vi "Write Array of Observer Refnum.vi"(8 "error in (no error)":errorcluster, 10 "Array of Observer Refnum":refnum<vi>, 11 "WT1600 in":refnum<class "WT1600.lvclass">) -> (0 "error out":errorcluster, 3 "WT1600 out":refnum<class "WT1600.lvclass">)   [LabVIEW 2013, in "WT1600.lvlib" / "WT1600.lvclass"]
uses:
  WT1600.lvclass
  <vilib>/ActorFramework/Message Enqueuer/Message Enqueuer.lvclass
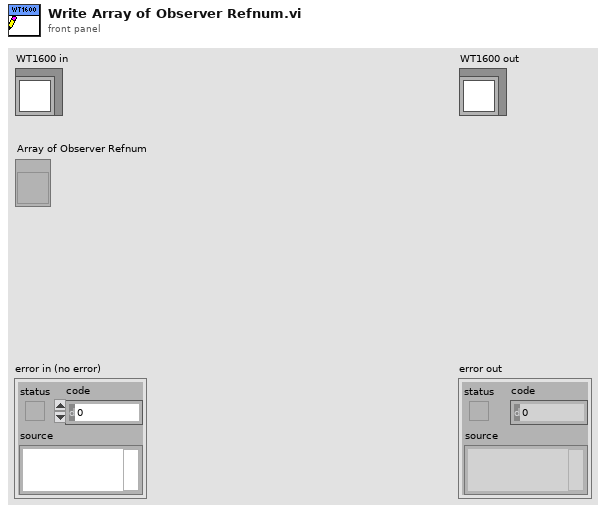
[diagram p1: front panel]
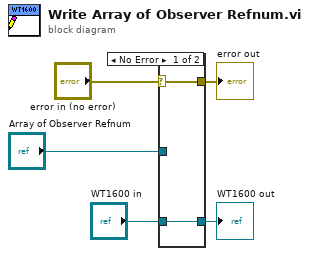
[diagram p0: block diagram]
diagram:
  n1 = case shown="No Error" "error in (no error)" {
    selector: "error in (no error)" -> [w7 w8]
    tunnel: [w7 w8] -> w4
    tunnel: [w6 w9] -> w2
    tunnel: "WT1600 in" -> [w6 w9]
    tunnel: "Array of Observer Refnum" -> [_ _]
    frame No Error {
    }
    frame Error {
    }
  }
  "error out" <- w4
  "WT1600 out" <- w2
